vi "test vision 2.vi"(3 "GIC Input":T1={"     Use ?\nOff       On"=[FALSE, TRUE, FALSE, TRUE], "Mode:"=FALSE, "Extra Port"="", "Hokuyo Port"="COM7", "Tx Prop  Port"="COM6", "Compass Port"="", "GPS Port"="", "Num of WPs"=0, "WP Lats and Longs"={"WP Lats"=[], "WP Longs"=[]}, "Obst Lats and Longs"={"Obst Lats"=[], "Obst Longs"=[]}, "Parameters"=[], "GPS Data"=[], "Compass"=0.0, "LMS Vector"=[], "Vision Vector"=[], "Direction Cmd"=0.0, "Speed Cmd"=0.0, "WP Vector"=[], "WP Number"=0, "Extra"=0, "SW Map"=[], "Path Cluster"={"Path x node"=[], "Path y node"=[]}, "Sim Course"=[]} {"Obst Lats and Longs"."Obst Longs" format="%#_8g"; "Obst Lats and Longs"."Obst Lats" format="%#_8g"}) -> (1 "GIC Output":T1={"     Use ?\nOff       On"=[FALSE, TRUE, FALSE, TRUE], "Mode:"=FALSE, "Extra Port"="", "Hokuyo Port"="COM7", "Tx Prop  Port"="COM6", "Compass Port"="", "GPS Port"="", "Num of WPs"=0, "WP Lats and Longs"={"WP Lats"=[], "WP Longs"=[]}, "Obst Lats and Longs"={"Obst Lats"=[], "Obst Longs"=[]}, "Parameters"=[], "GPS Data"=[], "Compass"=0.0, "LMS Vector"=[], "Vision Vector"=[], "Direction Cmd"=0.0, "Speed Cmd"=0.0, "WP Vector"=[], "WP Number"=0, "Extra"=0, "SW Map"=[], "Path Cluster"={"Path x node"=[], "Path y node"=[]}, "Sim Course"=[]} {"Obst Lats and Longs"."Obst Longs" format="%#_8g"; "Obst Lats and Longs"."Obst Lats" format="%#_8g"})   [LabVIEW 2014]
panel:
  out "out":dbl[][](array[numeric])
  in  "Green or Sat Max":dbl(slide)=84.70890410958904 scale=0.0..255.0
  in  "Blue or Luma Max":dbl(slide)=224.43493150684932 scale=0.0..255.0
  in  "Red or Hue Max":dbl(slide)=255.0 scale=0.0..255.0
  in  "Green or Sat Min":dbl(slide) scale=0.0..255.0
  in  "Blue or Luma Min":dbl(slide)=53.27054794520548 scale=0.0..255.0
  in  "Red or Hue Min":dbl(slide)=99.55479452054794 scale=0.0..255.0
  out "image out 2":T2(plugin-control)
  out "loop time":dbl=48.0
  in  "Stop (F)":bool
  out "image out":T2(plugin-control)
  # "Input:"
  # "Output:"
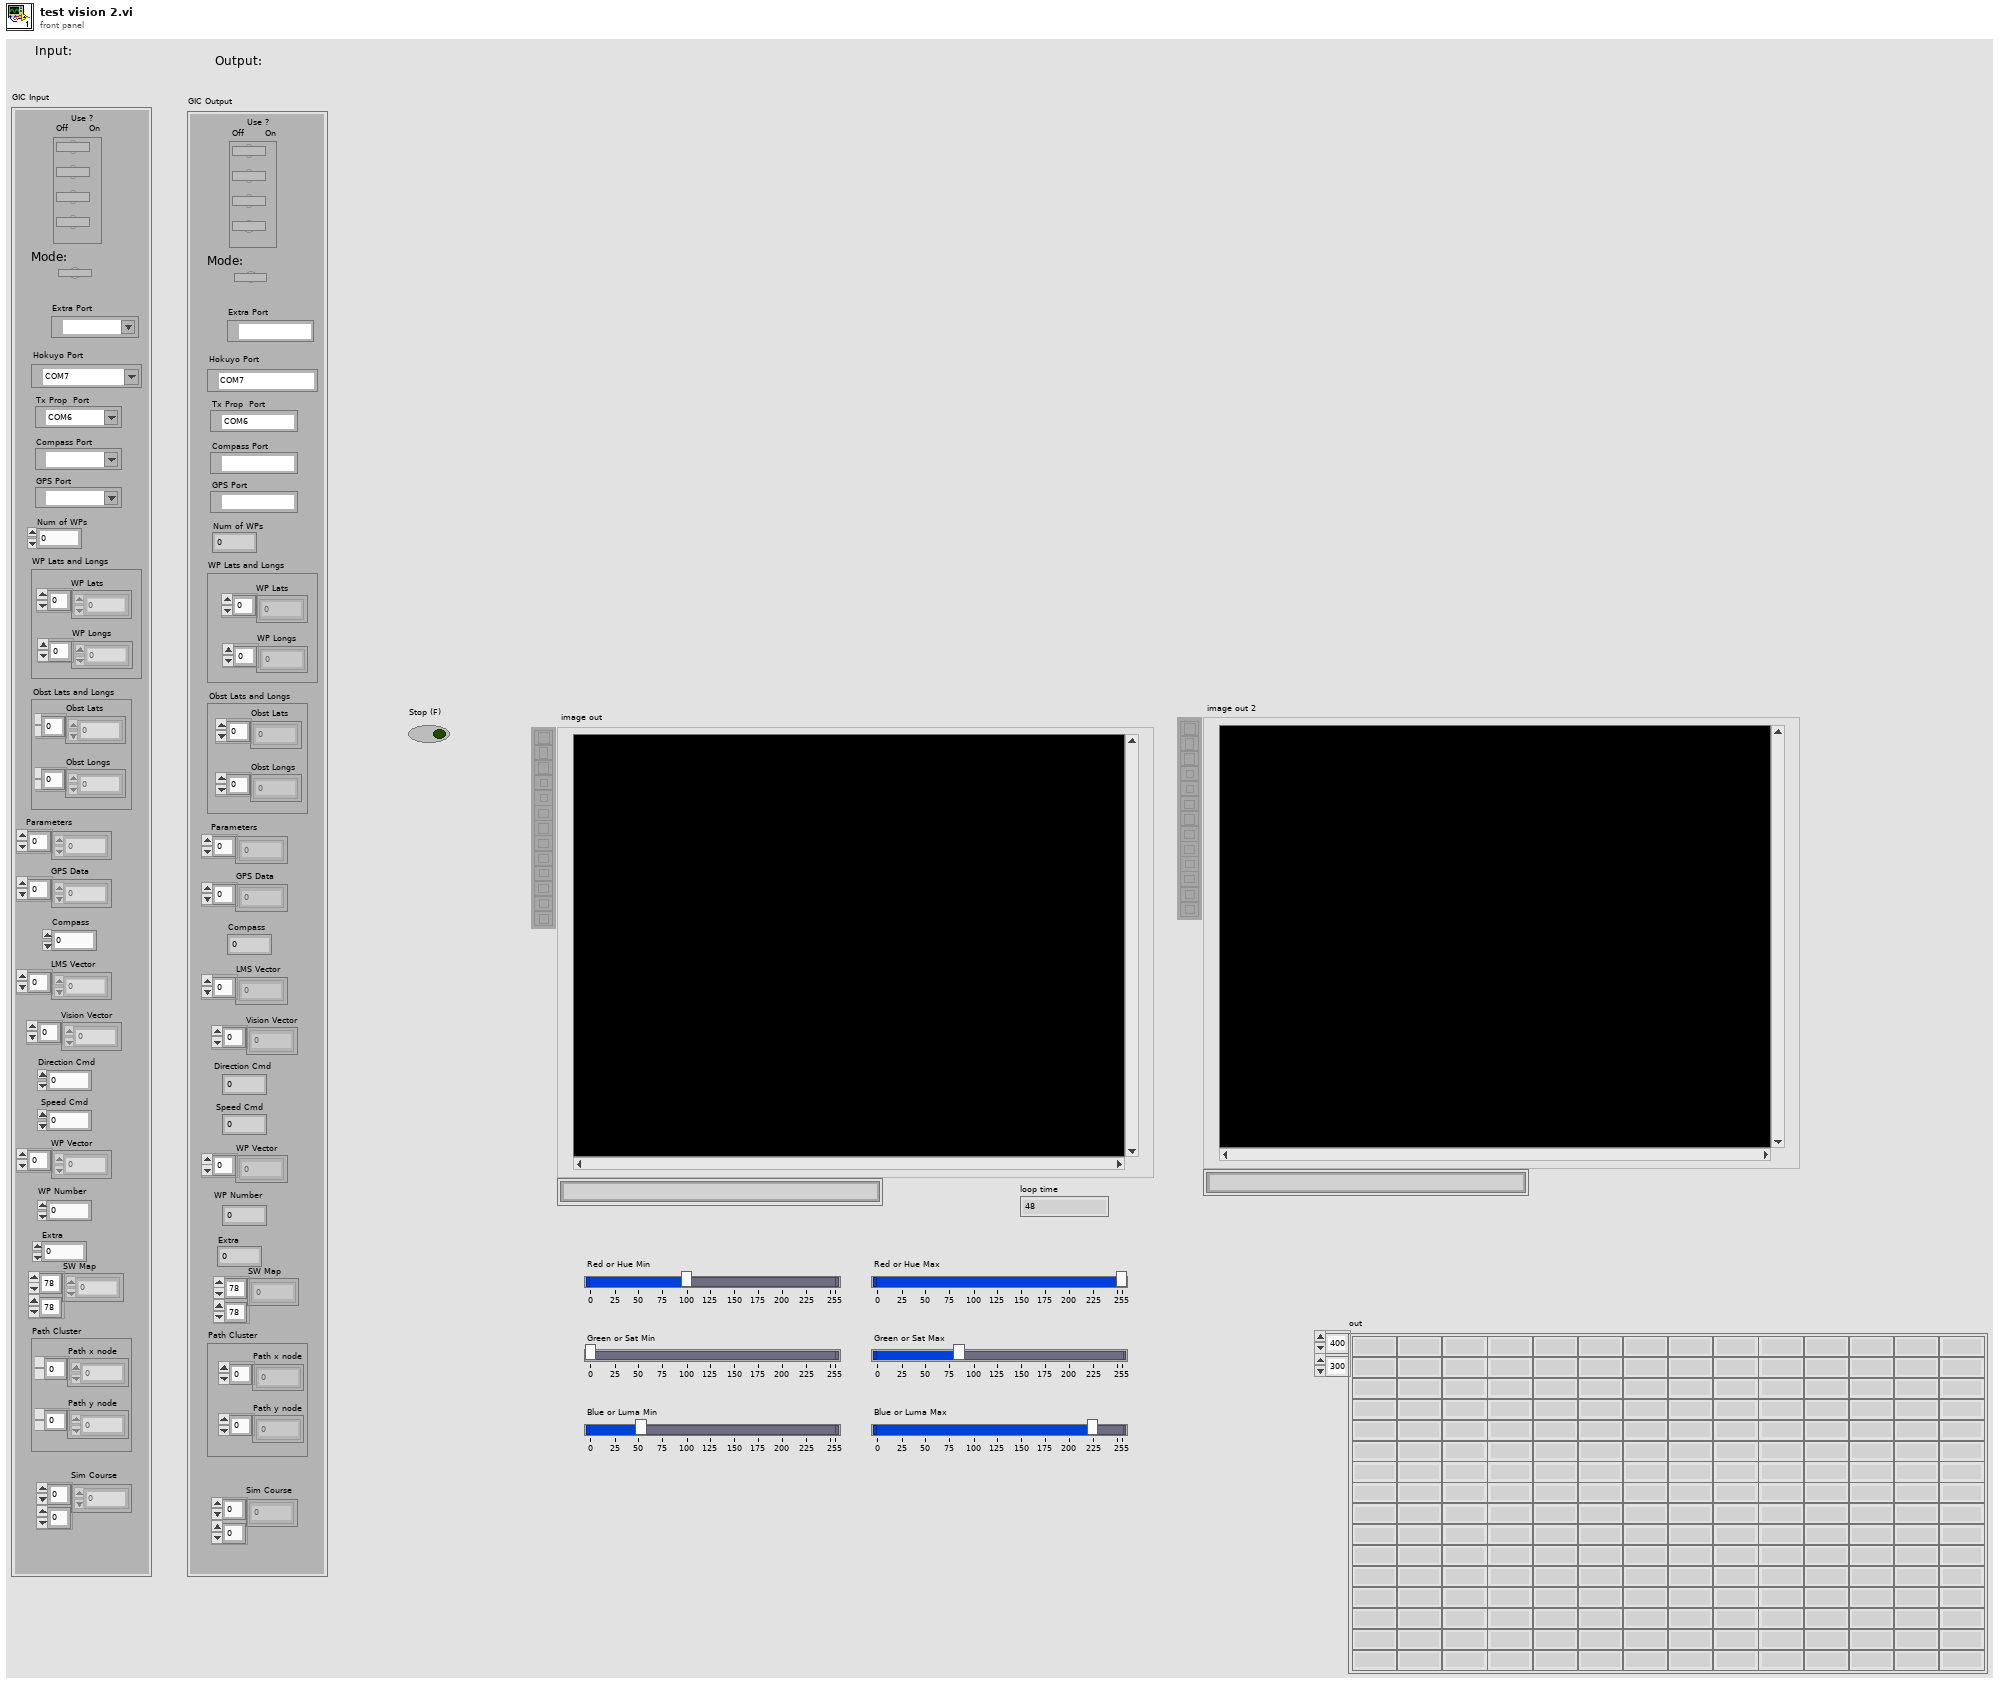
[diagram p1: front panel]
types:
  T1 = cluster{"     Use ?\nOff       On":bool[], "Mode:":bool, "Extra Port":refnum<visa-resource-name>, "Hokuyo Port":refnum<visa-resource-name>, "Tx Prop  Port":refnum<visa-resource-name>, "Compass Port":refnum<visa-resource-name>, "GPS Port":refnum<visa-resource-name>, "Num of WPs":i16, "WP Lats and Longs":cluster{"WP Lats":dbl[], "WP Longs":dbl[]}, "Obst Lats and Longs":cluster{"Obst Lats":dbl[], "Obst Longs":dbl[]}, "Parameters":dbl[], "GPS Data":dbl[], "Compass":dbl, "LMS Vector":dbl[], "Vision Vector":dbl[], "Direction Cmd":dbl, "Speed Cmd":dbl, "WP Vector":dbl[], "WP Number":i32, "Extra":i16, "SW Map":i32[][], "Path Cluster":cluster{"Path x node":dbl[], "Path y node":dbl[]}, "Sim Course":i8[][]}
  T2 = typedef "IMAQ Image.ctl" = refnum<image>
  T3 = cluster{"Red or Hue Min":dbl, "Red or Hue Max":dbl}
  T4 = cluster{"Green or Sat Min":dbl, "Green or Sat Max":dbl}
  T5 = cluster{"Blue or Luma Min":dbl, "Blue or Luma Max":dbl}
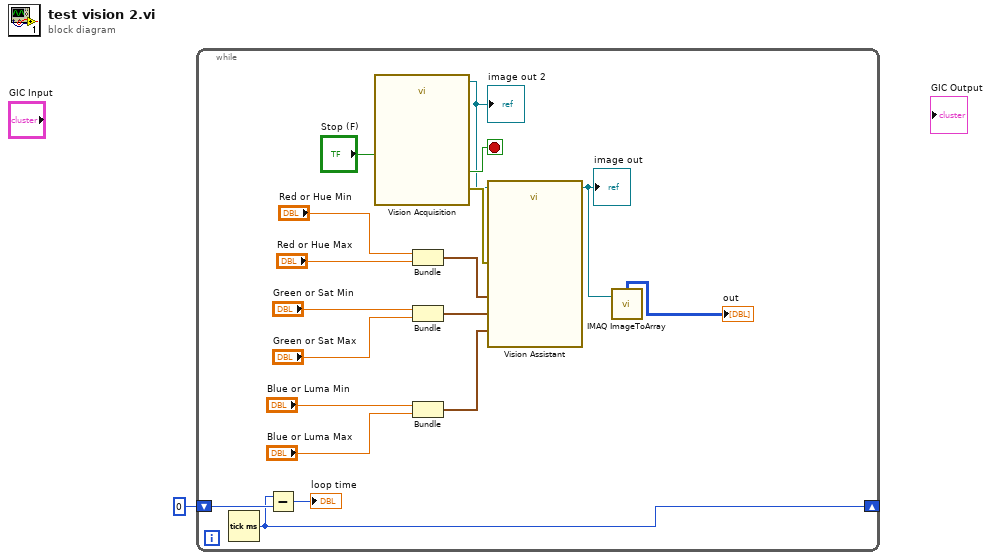
[diagram p0: block diagram]
diagram:
  n1 = while {
    shift-right: [w14] -> _
    shift-left: 0 -> [w16]
    stop <- w18 stop-if-true
    n2 = Tick Count (ms)() -> (millisecond timer value=w14:u32)
    n3 = Subtract(x=w14, y=w16) -> (x-y=→"loop time":u32)
    n4 = call "Vision Acquisition"("Stop (F)"="Stop (F)") -> ("Image Out"=w13:T2, "Stopped"=w18:bool, "error out"=w17:errorcluster)  [unwired: 24 in]
    "image out 2" <- w13
    n5 = Bundle("Red or Hue Min"="Red or Hue Min", "Red or Hue Max"="Red or Hue Max") -> (w10:T3)  [unwired: 1 in]
    n6 = Bundle("Green or Sat Min"="Green or Sat Min", "Green or Sat Max"="Green or Sat Max") -> (w7:T4)  [unwired: 1 in]
    n7 = Bundle("Blue or Luma Min"="Blue or Luma Min", "Blue or Luma Max"="Blue or Luma Max") -> (w4:T5)  [unwired: 1 in]
    n8 = call "Vision Assistant"("Image In"=w13, "Red or Hue Range (Color Threshold 1)"=w10, "Green or Sat Range (Color Threshold 1)"=w7, "Blue or Luma or Val or Inten Range (Color Threshold 1)"=w4, "error in"=w17) -> ("Image Out"=w3:T2)  [unwired: 21 in, 1 out]
    "image out" <- w3
    n9 = call "IMAQ ImageToArray"("Image"=w3) -> ("Image Pixels (U8)"=→"out":u8[][])  [unwired: 3 in, 4 out]
  }
